vi "HEWH Save Correct Condition.vi"(8 "Error In":errorcluster, 10 "Current Cond":T1, 11 "Saved Condition":T1) -> (0 "Error Out":errorcluster, 3 "Saved Condition Read":T1)   [LabVIEW 2020]
uses:
  Type Definitions/HEWH Special Condition Check.ctl
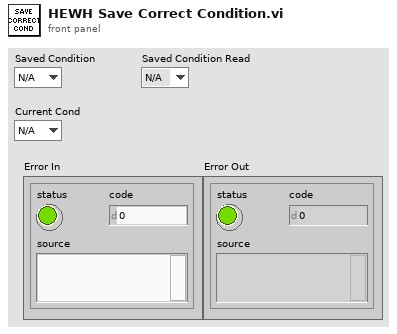
[diagram p1: front panel]
types:
  T1 = typedef "HEWH Special Condition Check.ctl" = enum16{"N/A", "C1", "C2", "Reset/Fail", "Skip Draw Sequence"}
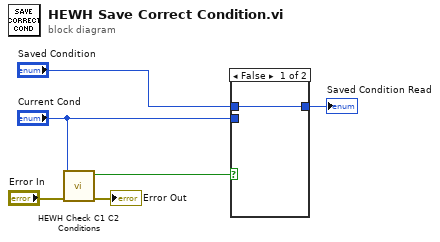
[diagram p0: block diagram]
diagram:
  n1 = call "HEWH Check C1 C2 Conditions.vi"("Error In"="Error In", "Current Input"="Current Cond") -> ("Error Out"=→"Error Out":errorcluster, "C1 or C2?"=w3:bool)  [unwired: 8 in]
  n2 = case shown="False" w3 {
    tunnel: "Current Cond" -> [_ w8]
    tunnel: [w7 w8] -> w4
    tunnel: "Saved Condition" -> [w7 _]
    frame False {
    }
    frame True {
    }
  }
  "Saved Condition Read" <- w4
